vi "MM6.ProcConstructor.vi"(0 "i ref in":refnum<vi>, 3 "ms timeout (10000)":i32=10000, 5 "error in (no error)":errorcluster) -> (14 "i ref out":refnum<vi>, 19 "error out":errorcluster)   [LabVIEW 2014, in "MM6.lvlib"]
doc: "This method allows to do initialization (to serve as a constructor for attributes). It is necessary, since the BaseProcess.i attribute is not initialized when the ClassName.constructor is executed."
uses:
  MM6.lvlib
  MM6.status.ctl
  CSCore/CSSystem/CoreLib/CoreLib.string 2 byte array.vi
  CSCore/BaseProcess/BaseProcess.lvlib
  CSCore/CSSystem/CSSystemLib/CSSystemLib.lvlib
  CSCore/CSSystem/CoreLib/CoreLib.lvlib
  CSlibraries-extern/DimLVEvent/LVDimInterface/LVDimInterface.lvlib
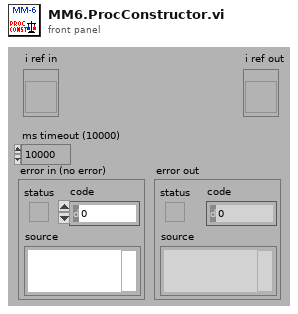
[diagram p1: front panel]
types:
  T1 = typedef "MM6.lvlib/MM6.status.ctl" = enum16{"loaded", "load_error", "config", "config_error", "init", "init_error", "data_reset", "data_reset_error", "running", "start_error", "run_error", "abort_requested", "aborted", "stop_requested", "stopped", "stop_error", "Connected", "NOTConnected"}
  T2 = typedef "CoreDefs.rawDataType.ctl" = i8[]
  T3 = typedef "MM6.lvlib/MM6.i attribute.ctl" = cluster{"ConfigData":T4, "UsedObjs":string[], "ActScanStep":i32[], "AbortRequest":bool, "StopRequest":bool, "# cycles":i32, "Connected":bool, "MMStatus":T1, "# data":i32, "DIMServices":cluster{"MM6StatusString":string, "MM6StatusID":i32, "discArchiver":string, "discArchiverID":i32, "eventBuilder":string, "eventBuilderID":i32, "GUIIDString":string, "GUIIDStringID":i32}, "dataFile":string, "ExtraDataSets":T19, "PGRunning":T20}
  T4 = typedef "LEBITDefs.lvlib/LEBITDefs.ConfigData.ctl" = cluster{"GenConfig":T5, "Configs":T7[]}
  T5 = typedef "LEBITDefs.lvlib/LEBITDefs.GenConfig.ctl" = cluster{"Mode":i32, "Logs":T6[]}
  T6 = typedef "LEBITDefs.lvlib/LEBITDefs.Log.ctl" = cluster{"Name":string, "FctName":string, "Special":string}
  T7 = typedef "LEBITDefs.lvlib/LEBITDefs.OneConfig.ctl" = cluster{"MCA":T8, "Timing":T9, "Scans":T12[], "FreqDevs":T13[], "CleanDev":T14, "NrCycles":i32, "Specials":T16[], "Delays":T17[], "DAC":T18}
  T8 = typedef "LEBITDefs.lvlib/LEBITDefs.MCA.ctl" = cluster{"Name":string, "Address":string, "NrChannels":i32, "Gate":i32, "NrPipse":i32}
  T9 = typedef "LEBITDefs.lvlib/LEBITDefs.Timing.ctl" = cluster{"TimeTables":cluster{"TimeTable":T10}[], "Memories":T11[], "ScanX":string, "ScanY":string}
  T10 = typedef "LEBITDefs.lvlib/LEBITDefs.Timetable.ctl" = dbl[]
  T11 = typedef "LEBITDefs.lvlib/LEBITDefs.Memory.ctl" = cluster{"Device":string, "ExtTrig":bool, "TT2Use":i32, "PatternTable":string[]}
  T12 = typedef "LEBITDefs.lvlib/LEBITDefs.ScanDev.ctl" = cluster{"Name":string, "FctName":string, "Values":dbl[], "NrScanVals":i32, "Special":string}
  T13 = typedef "LEBITDefs.lvlib/LEBITDefs.FreqDev.ctl" = cluster{"Name":string, "Amp":dbl, "CenterFreq":dbl, "Time":dbl}
  T14 = typedef "LEBITDefs.lvlib/LEBITDefs.CleanDev.ctl" = cluster{"Name":string, "CleanData":T15[]}
  T15 = typedef "LEBITDefs.lvlib/LEBITDefs.CleanDataType.ctl" = cluster{"Amp":dbl, "Center":dbl, "Plus":dbl, "Minus":dbl, "Time":dbl}
  T16 = typedef "LEBITDefs.lvlib/LEBITDefs.Special.ctl" = cluster{"Name":string, "FctName":string, "VerySpecial":string, "Data":dbl}
  T17 = typedef "LEBITDefs.lvlib/LEBITDefs.Delay.ctl" = cluster{"Name":string, "Delay":dbl}
  T18 = typedef "LEBITDefs.lvlib/LEBITDefs.DAC.ctl" = cluster{"Name":string, "Step1":i32, "Step2":i32}
  T19 = typedef "LEBITDefs.lvlib/LEBITDefs.ExtraData.ctl" = cluster{"Ions":cluster{"ExcitIonMass":string, "ExcitIonCharge":i32, "CleanIons":cluster{"CleanIonMass":string, "CleanIonCharge":i32}[]}, "TimingDescription":cluster{"TimeTableDescription":cluster{"Times":string[]}[], "PatternTableDescription":cluster{"Pattern":string[]}[]}, "ScanUnits":string[]}[]
  T20 = typedef "PPG_ABC.lvlib/PPG_ABC.PG_Running.ctl" = i32
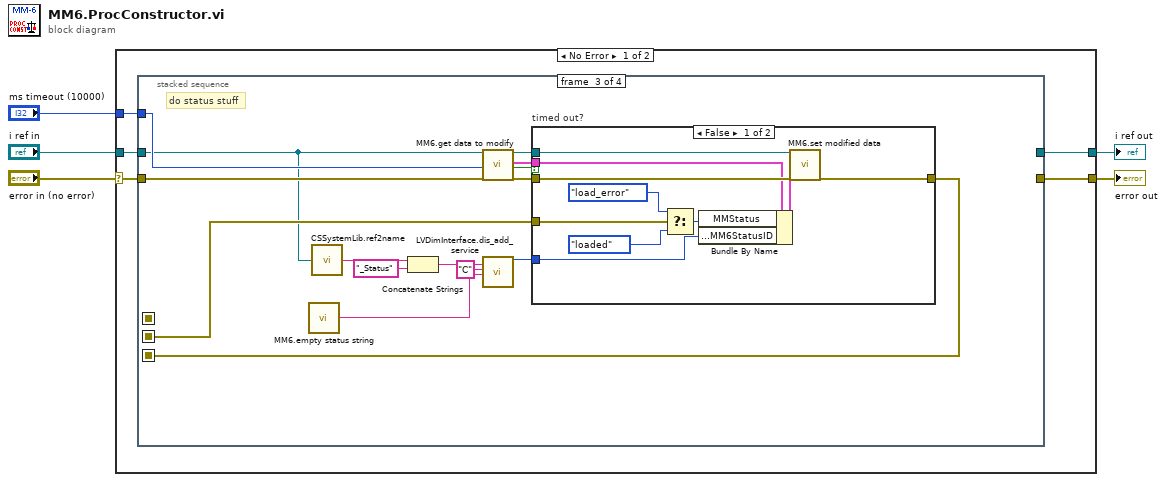
[diagram p0: block diagram]
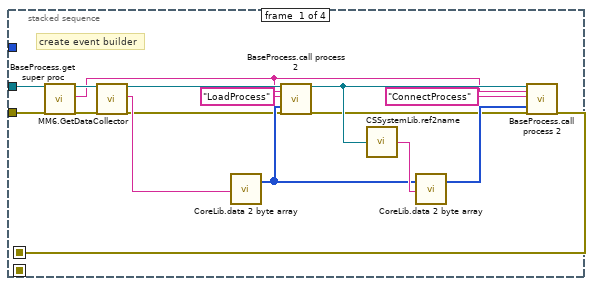
[diagram p2: hidden frame]
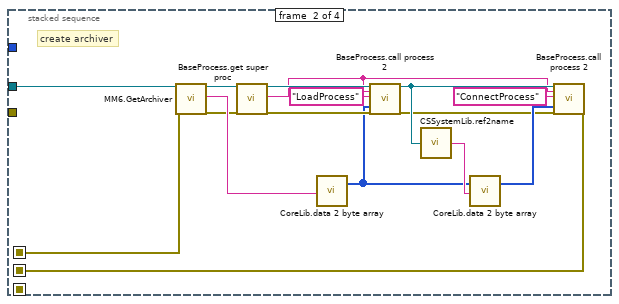
[diagram p3: hidden frame]
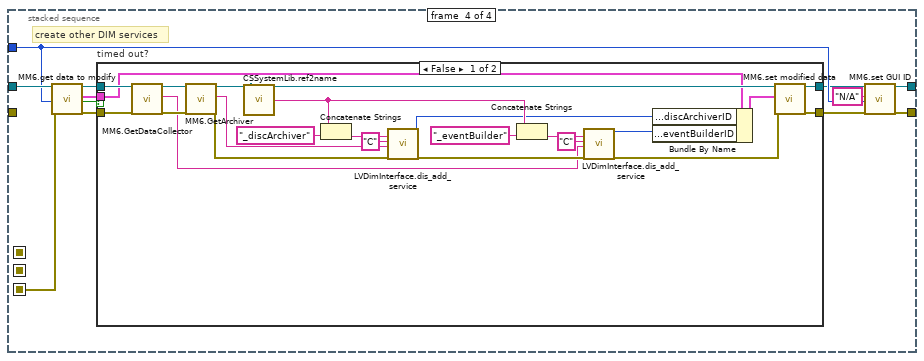
[diagram p5: hidden frame]
diagram:
  n1 = case shown="No Error" "error in (no error)" {
    selector: "error in (no error)" -> [w6 w106]
    tunnel: [w10 w107] -> w5
    tunnel: [w9 w106] -> w4
    tunnel: "i ref in" -> [w8 w107]
    tunnel: "ms timeout (10000)" -> [w7 _]
    frame No Error {
      n2 = stacked-sequence {
        seq-local: [w19 _ _ _] -> [_ w40 _ _]
        seq-local: [_ w27 _ _] -> [_ _ w52 _]
        seq-local: [_ _ w43 _] -> [_ _ _ w71]
        tunnel: w8 -> [w24 w41 w50 w80]
        tunnel: w6 -> [w11 _ w54 _]
        tunnel: w7 -> [_ _ w51 w75]
        tunnel: [_ _ _ w69] -> w10
        tunnel: [_ _ _ w70] -> w9
        frame #0 {
          # "create event builder"
          n3 = call "BaseProcess.get super proc.vi"("i ref in"=w24, "error in (no error)"=w11) -> ("i ref out"=w26:refnum<vi>, "SuperProc"=w16:string, "error out"=w25:errorcluster)  [unwired: 15 in]
          n4 = call "MM6.GetDataCollector.vi"("i ref in"=w26, "error in (no error)"=w25) -> ("i ref out"=w18:refnum<vi>, "data collector"=w20:string, "error out"=w13:errorcluster)  [unwired: 15 in]
          n5 = call-poly "CoreLib.data 2 byte array.vi"("string"=w20) -> ("byteArray out"=w14:T2)  [unwired: 18 in]
          n6 = call "BaseProcess.call process 2.vi"("i ref in"=w18, "Object"=w16, "Selector"="LoadProcess", "Data"=w14, "error in (no error)"=w13) -> ("i ref out"=w17:refnum<vi>, "error out"=w12:errorcluster)  [unwired: 13 in]
          n7 = call "CSSystemLib.ref2name.vi"("obj refnum"=w17) -> ("name"=w22:string)
          n8 = call-poly "CoreLib.data 2 byte array.vi"("byteArray"=w14, "string"=w22) -> ("byteArray out"=w21:T2)  [unwired: 17 in]
          n9 = call "BaseProcess.call process 2.vi"("i ref in"=w17, "Object"=w16, "Selector"="ConnectProcess", "Data"=w21, "error in (no error)"=w12) -> ("error out"=w19:errorcluster)  [unwired: 13 in, 1 out]
        }
        frame #1 {
          # "create archiver"
          n10 = call "MM6.GetArchiver.vi"("i ref in"=w41, "error in (no error)"=w40) -> ("i ref out"=w38:refnum<vi>, "archiver"=w42:string, "error out"=w39:errorcluster)  [unwired: 15 in]
          n11 = call "BaseProcess.get super proc.vi"("i ref in"=w38, "error in (no error)"=w39) -> ("i ref out"=w34:refnum<vi>, "SuperProc"=w30:string, "error out"=w32:errorcluster)  [unwired: 15 in]
          n12 = call-poly "CoreLib.data 2 byte array.vi"("string"=w42) -> ("byteArray out"=w28:T2)  [unwired: 18 in]
          n13 = call "BaseProcess.call process 2.vi"("i ref in"=w34, "Object"=w30, "Selector"="LoadProcess", "Data"=w28, "error in (no error)"=w32) -> ("i ref out"=w33:refnum<vi>, "error out"=w31:errorcluster)  [unwired: 13 in]
          n14 = call "CSSystemLib.ref2name.vi"("obj refnum"=w33) -> ("name"=w36:string)
          n15 = call-poly "CoreLib.data 2 byte array.vi"("byteArray"=w28, "string"=w36) -> ("byteArray out"=w35:T2)  [unwired: 17 in]
          n16 = call "BaseProcess.call process 2.vi"("i ref in"=w33, "Object"=w30, "Selector"="ConnectProcess", "Data"=w35, "error in (no error)"=w31) -> ("error out"=w27:errorcluster)  [unwired: 13 in, 1 out]
        }
        frame #2 {
          # "do status stuff"
          n17 = call "MM6.empty status string.vi"() -> ("String"=w44:string)
          n18 = call "CSSystemLib.ref2name.vi"("obj refnum"=w50) -> ("name"=w49:string)
          n19 = Concatenate Strings(w49, "_Status" ("string")) -> (w47:string)
          n20 = call "MM6.get data to modify.vi"("i ref in"=w50, "ms timeout (10000)"=w51, "error in (no error)"=w54) -> ("i ref out"=w57:refnum<vi>, "i attribute"=w56:T3, "timed out"=w55:bool, "error out"=w53:errorcluster)  [unwired: 13 in]
          n21 = call "LVDimInterface.dis_add_service.vi"("serviceName"=w47, "typeDescriptor"="C", "data"=w44) -> ("my_serviceID"=w45:i32)  [unwired: 15 in, 1 out]
          n22 = case "timed out?" shown="False" w55 {
            tunnel: w57 -> [w67 _]
            tunnel: w56 -> [w65 _]
            tunnel: w53 -> [w66 w68]
            tunnel: w52 -> [w63 _]
            tunnel: [w59 w68] -> w43
            tunnel: w45 -> [w58 _]
            frame False {
              n23 = Select(t=MM6.status."load_error" ("MMStatus"), s=w63, f=MM6.status."loaded" ("MMStatus")) -> (s? t:f=w60:T1)
              n24 = Bundle By Name(cluster=w65, "MMStatus"=w60, "DIMServices.MM6StatusID"=w58) -> (w64:T3)
              n25 = call "MM6.set modified data.vi"("i ref in"=w67, "i attribute"=w64, "error in (no error)"=w66) -> ("error out"=w59:errorcluster)  [unwired: 15 in, 1 out]
            }
            frame True {
            }
          }
        }
        frame #3 {
          # "create other DIM services"
          n26 = call "MM6.get data to modify.vi"("i ref in"=w80, "ms timeout (10000)"=w75, "error in (no error)"=w71) -> ("i ref out"=w78:refnum<vi>, "i attribute"=w76:T3, "timed out"=w79:bool, "error out"=w77:errorcluster)  [unwired: 13 in]
          n27 = case "timed out?" shown="False" w79 {
            tunnel: w78 -> [w103 w105]
            tunnel: w77 -> [w99 w104]
            tunnel: w76 -> [w87 _]
            tunnel: [w82 w105] -> w74
            tunnel: [w81 w104] -> w73
            frame False {
              n28 = call "MM6.GetDataCollector.vi"("i ref in"=w103, "error in (no error)"=w99) -> ("i ref out"=w102:refnum<vi>, "data collector"=w89:string, "error out"=w101:errorcluster)  [unwired: 15 in]
              n29 = call "MM6.GetArchiver.vi"("i ref in"=w102, "error in (no error)"=w101) -> ("i ref out"=w100:refnum<vi>, "archiver"=w95:string, "error out"=w94:errorcluster)  [unwired: 15 in]
              n30 = call "CSSystemLib.ref2name.vi"("obj refnum"=w100) -> ("name"=w88:string)
              n31 = Concatenate Strings(w88, "_discArchiver" ("string")) -> (w97:string)
              n32 = call "LVDimInterface.dis_add_service.vi"("serviceName"=w97, "typeDescriptor"="C", "data"=w95, "error in (no error)"=w94) -> ("my_serviceID"=w85:i32, "error out"=w90:errorcluster)  [unwired: 14 in]
              n33 = Concatenate Strings(w88, "_eventBuilder" ("string")) -> (w92:string)
              n34 = call "LVDimInterface.dis_add_service.vi"("serviceName"=w92, "typeDescriptor"="C", "data"=w89, "error in (no error)"=w90) -> ("my_serviceID"=w84:i32, "error out"=w83:errorcluster)  [unwired: 14 in]
              n35 = Bundle By Name(cluster=w87, "DIMServices.discArchiverID"=w85, "DIMServices.eventBuilderID"=w84) -> (w86:T3)
              n36 = call "MM6.set modified data.vi"("i ref in"=w100, "i attribute"=w86, "error in (no error)"=w83) -> ("i ref out"=w82:refnum<vi>, "error out"=w81:errorcluster)  [unwired: 15 in]
            }
            frame True {
            }
          }
          n37 = call "MM6.set GUI ID.vi"("i ref in"=w74, "GUIDString"="N/A", "ms timeout (10000)"=w75, "error in (no error)"=w73) -> ("i ref out"=w69:refnum<vi>, "error out"=w70:errorcluster)  [unwired: 13 in, 1 out]
        }
      }
    }
    frame Error {
    }
  }
  "error out" <- w4
  "i ref out" <- w5
